vi "PhotonCamera_GetDriverMode.vi"(11 "CameraName":string) -> (3 "DriverMode":bool)   [LabVIEW 2019, in "PhotonVisionLib.lvlib"]
doc: "Returns whether the camera is in driver mode.\n\nInputs:\n - CameraName -- The nickname of the camera (found in the PhotonVision UI).\n \nOutputs:\n - DriverMode -- Boolean indicating whether the camera is in driver mode."
uses:
  PhotonVisionLib.lvlib
  <vilib>/Rock Robotics/Network Tables/NT Read Boolean.vi
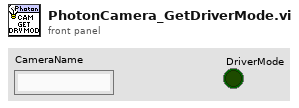
[diagram p1: front panel]
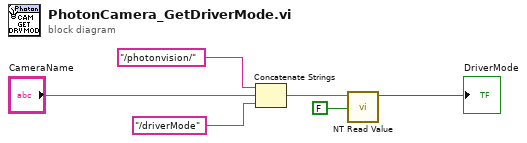
[diagram p0: block diagram]
diagram:
  n1 = Concatenate Strings("/photonvision/", "CameraName", "/driverMode") -> (w3:string)
  n2 = call-poly <vilib>:"NT Read Value.vi"("Default Value"=FALSE, "Name"=w3) -> ("Boolean"=→"DriverMode":bool)  [unwired: 8 in, 1 out]
